vi "Set Header Object Positions.vi"(8 "error in":errorcluster, 10 "label array in":string[](array[string]), 11 "controls[] in":refnum<vi>[](array[refnum])) -> (0 "error out":errorcluster, 2 "label array out":string[](array[string]), 3 "controls[] out":refnum<vi>[](array[refnum]))   [LabVIEW 2018]
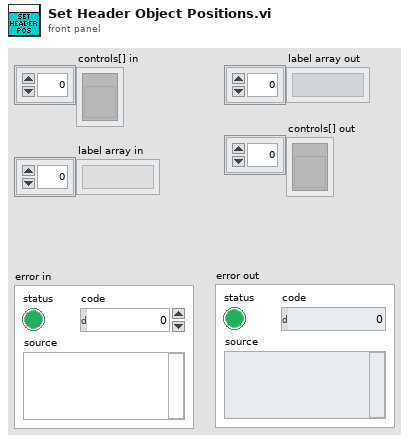
[diagram p1: front panel]
types:
  T1 = typedef "LVRectTypeDef.ctl" = cluster{"Left":i16, "Top":i16, "Right":i16, "Bottom":i16}
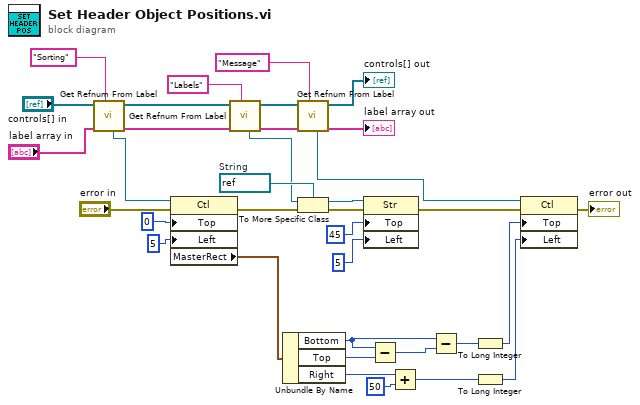
[diagram p0: block diagram]
diagram:
  w27 = refnum<vi> refnum  # String
  n1 = call "Get Refnum From Label.vi"("label"="Sorting" ("element"), "label array in"="label array in", "controls[] in"="controls[] in") -> ("label array out"=w8:string[], "controls[] out"=w7:refnum<vi>[], "refnum out"=w9:refnum<vi>)  [unwired: 6 in]
  n2 = property class="Ctl"(reference=w9, error in="error in", "Top"=0 ("Position:Left"), "Left"=5 ("Position:Top")) -> (error out=w30:errorcluster, "MasterRect"=w22:T1)  [unwired: 1 out]
  n3 = call "Get Refnum From Label.vi"("label"="Labels" ("element"), "label array in"=w8, "controls[] in"=w7) -> ("label array out"=w32:string[], "controls[] out"=w33:refnum<vi>[], "refnum out"=w26:refnum<vi>)  [unwired: 6 in]
  n4 = Unbundle By Name(w22) -> ("Bottom"=w23:i16, "Top"=w15:i16, "Right"=w17:i16)
  n5 = call "Get Refnum From Label.vi"("label"="Message", "label array in"=w32, "controls[] in"=w33) -> ("label array out"=→"label array out":string[], "controls[] out"=→"controls[] out":refnum<vi>[], "refnum out"=w16:refnum<vi>)  [unwired: 6 in]
  n6 = To More Specific Class(target class=w27, reference=w26, error in=w30) -> (specific class reference=w28:refnum<vi>, error out=w31:errorcluster)
  n7 = property class="Str"(reference=w28, error in=w31, "Top"=45 ("Position:Top"), "Left"=5 ("Position:Left")) -> (error out=w2:errorcluster)  [unwired: 1 out]
  n8 = Subtract(x=w23, y=w15) -> (x-y=w24:i16)
  n9 = Add(x=w17, y=i16 50) -> (x+y=w20:i16)
  n10 = Subtract(x=w23, y=w24) -> (x-y=w25:i16)
  n11 = To Long Integer(number=w25) -> (32bit integer=w18:i32)
  n12 = To Long Integer(number=w20) -> (32bit integer=w19:i32)
  n13 = property class="Ctl"(reference=w16, error in=w2, "Top"=w18, "Left"=w19) -> (error out=→"error out":errorcluster)  [unwired: 1 out]
